vi "Write SHV SM Ticks.vi"(8 "error in (no error)":errorcluster, 10 "Ticks (0)":i16, 11 "Stepper in":refnum<class "Stepper.lvclass">) -> (0 "error out":errorcluster, 3 "Stepper out":refnum<class "Stepper.lvclass">)   [LabVIEW 2015, in "Stepper.lvclass"]
uses:
  Stepper.lvclass
  Stepper.lvclass/Stepper.ctl
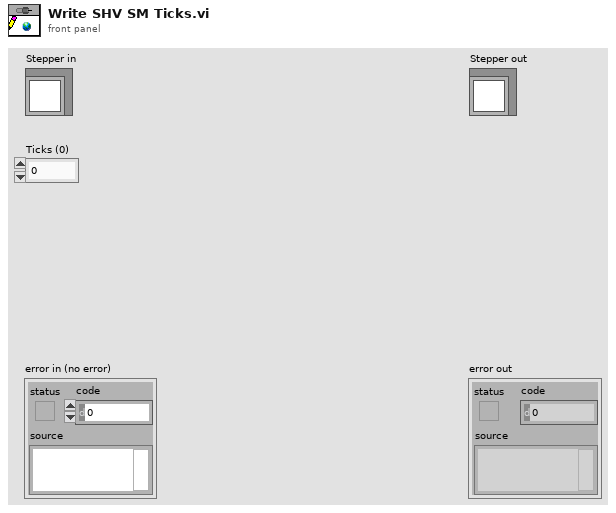
[diagram p1: front panel]
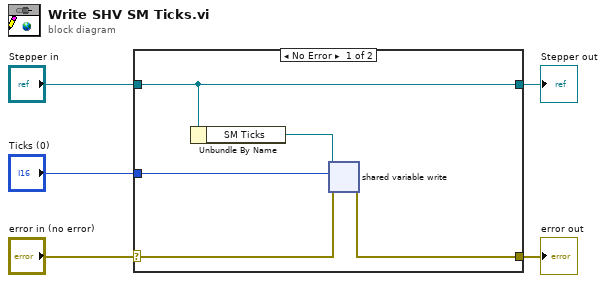
[diagram p0: block diagram]
diagram:
  n1 = case shown="No Error" "error in (no error)" {
    selector: "error in (no error)" -> [w7 w11]
    tunnel: [w6 w11] -> w4
    tunnel: [w10 w12] -> w2
    tunnel: "Stepper in" -> [w10 w12]
    tunnel: "Ticks (0)" -> [w8 _]
    frame No Error {
      n2 = Unbundle By Name(w10) -> ("SM Ticks"=w9:refnum<k21>)
      n3 = shared-variable-write(w9, w7, w8) -> (w6:errorcluster)  [unwired: 1 out]
    }
    frame Error {
    }
  }
  "error out" <- w4
  "Stepper out" <- w2
